vi "Compose LabVIEW Object - Interface - Returns No Error.vi"() -> ()   [LabVIEW 2020]
uses:
  92f102a0-c856-46da-bf7d-d489e92c860f.vi
  <vilib>/addons/_JKI Toolkits/Caraya/classes/Test/Test.lvclass
  <vilib>/addons/_JKI Toolkits/Caraya/classes/Assert/Assert.lvclass
  <vilib>/addons/_JKI Toolkits/Caraya/classes/Assert/Assert Not Error.vi
  IDisposable/IDisposable.lvclass
panel:
  out "LabVIEW Object":refnum<class "IDisposable.lvclass">
  out "error out":errorcluster
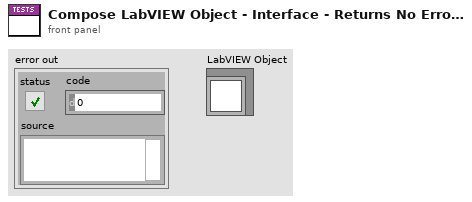
[diagram p1: front panel]
types:
  T1 = cluster{"Major":u16, "Minor":u16, "Fix":u16, "Build":u16}[]
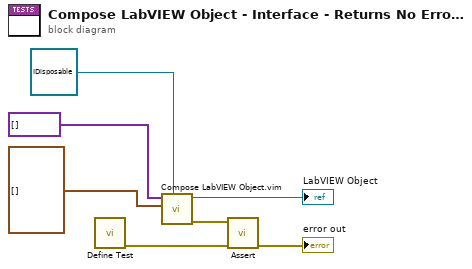
[diagram p0: block diagram]
diagram:
  n1 = call <vilib>:"Define Test.vi"() -> ("error out"=w4:errorcluster)  [unwired: 10 in, 1 out]
  n2 = call "Compose LabVIEW Object.vim"("Type"=refnum<class "IDisposable.lvclass"> refnum ("Reflection.Tests.lvlib:String.lvclass"), "Library Versions"=T1 [], "Private Data Clusters"=variant[] []) -> ("error out"=w5:errorcluster, "LabVIEW Object"=→"LabVIEW Object":refnum<class "IDisposable.lvclass">)  [unwired: 7 in]
  n3 = call-poly <vilib>:"Assert.vi"("error in (no error)"=w4, "Not Error?"=w5) -> ("error out"=→"error out":errorcluster)  [unwired: 8 in, 1 out]
